vi "Pre Launch Init.vi"(11 "Sim Sensor Interface Actor in":refnum<class "Sim Sensor Interface Actor.lvclass">) -> (0 "error out":errorcluster, 3 "Sim Sensor Interface Actor out":refnum<class "Sim Sensor Interface Actor.lvclass">)   [LabVIEW 2022 SP3, in "Sim Sensor Interface Actor.lvlib" / "Sim Sensor Interface Actor.lvclass"]
doc: "(<B>Filename</B>: Actor Framework.lvlib:Actor.lvclass:Pre Launch Init.vi)\n\nDefines behavior that occurs after the Launch Actor method is invoked but before the actor's Actor Core method begins running.\n\nThe Pre Launch Init method is guaranteed to finish before the Launch Actor method returns to its caller and before the actor itself receives any messages. Any references that the Pre Launch Init method obtains are guaranteed to have the same lifetime as the actor itself. Any errors that the Pre Launch Init method returns will abort the launch.\n\nBy default, this method does nothing. A descendant class may override it to define behavior."
uses:
  Sim Sensor Interface Actor.lvclass
  Sim Sensor Interface Actor.lvclass/Sim Sensor Interface Actor.ctl
  Abstract Sensor Interface Actor/Abstract Sensor Interface Actor/Abstract Sensor Interface Actor.lvclass
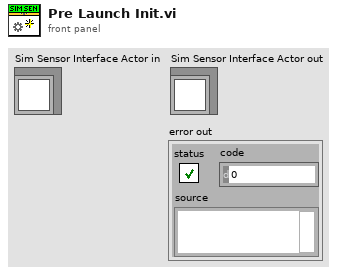
[diagram p1: front panel]
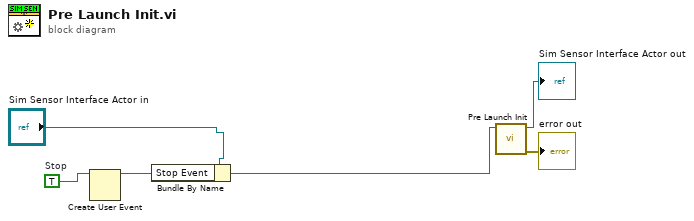
[diagram p0: block diagram]
diagram:
  w3 = TRUE  # Stop
  n1 = Create User Event(user event datatype=w3) -> (user event=w4:refnum<user-event>)  [unwired: 1 in, 1 out]
  n2 = Bundle By Name(cluster="Sim Sensor Interface Actor in", "Stop Event"=w4) -> (w1:refnum<class "Sim Sensor Interface Actor.lvclass">)
  n3 = call-parent "Pre Launch Init.vi"("Actor in"=w1) -> ("error out"=→"error out":errorcluster, "Actor out"=→"Sim Sensor Interface Actor out":refnum<class "Sim Sensor Interface Actor.lvclass">)  [unwired: 9 in]
